vi "randomgraph.vi"() -> ()   [LabVIEW 2019]
panel:
  in  "?":bool
  in  "Save To Excel":bool
  out "Waveform Graph":dbl[][](graph)
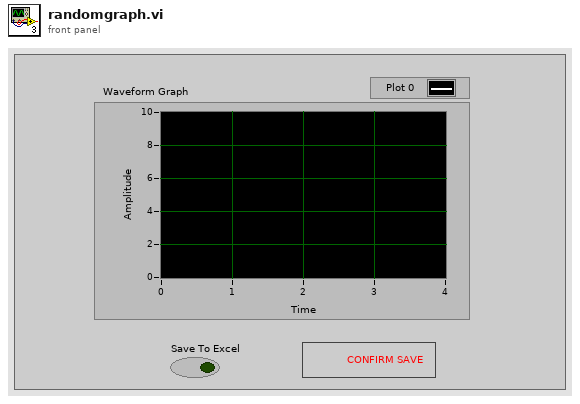
[diagram p1: front panel]
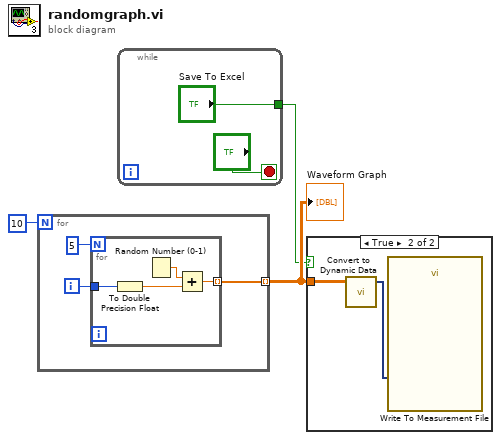
[diagram p0: block diagram]
diagram:
  n1 = for {
    N: 10 -> [_]
    tunnel: [w4] -> w2 mode=indexing
    i -> [w5]
    n2 = for {
      N: 5 -> [_]
      tunnel: [w10] -> w4 mode=indexing
      tunnel: w5 -> [w8]
      n3 = To Double Precision Float(number=w8) -> (double precision float=w7:dbl)
      n4 = Random Number (0-1)() -> (number: 0 to 1=w9:dbl)
      n5 = Add(x=w9, y=w7) -> (x+y=w10:dbl)
    }
  }
  "Waveform Graph" <- w2
  n6 = while {
    tunnel: ["Save To Excel"] -> w1
    stop <- "?" stop-if-true
  }
  n7 = case shown="True" w1 {
    tunnel: w2 -> [_ w14]
    frame False {
    }
    frame True {
      n8 = call "Convert to Dynamic Data"("2D Array"=w14) -> ("Dynamic Data Type"=w13:dynamicdata)  [unwired: 3 in]
      n9 = call "Write To Measurement File"("Signals"=w13) -> ()  [unwired: 16 in, 3 out]
    }
  }
